vi "10.6.vi"() -> ()   [LabVIEW 2019]
panel:
  out "Numeric":dbl
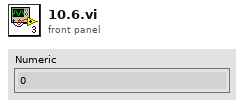
[diagram p1: front panel]
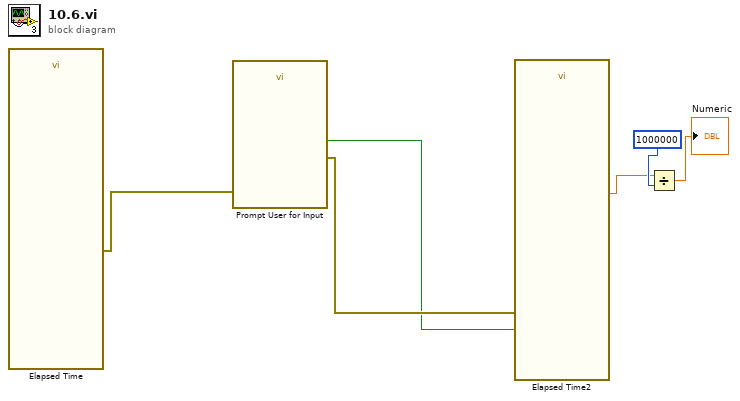
[diagram p0: block diagram]
diagram:
  n1 = call "Elapsed Time"() -> ("error out"=w6:errorcluster)  [unwired: 12 in, 7 out]
  n2 = call "Prompt User for Input"("error in (no error)"=w6) -> ("OK"=w4:bool, "error out"=w5:errorcluster)  [unwired: 17 in]
  n3 = call "Elapsed Time2"("Reset"=w4, "error in (no error)"=w5) -> ("Present (s)"=w1:dbl)  [unwired: 10 in, 7 out]
  n4 = Divide(x=w1, y=1000000) -> (x/y=→"Numeric":dbl)
